vi "Read Set.vi"(8 "error in (no error)":errorcluster, 11 "VISA resource name":refnum<visa-resource-name>) -> (0 "error out":errorcluster, 1 "Set Current Level (A)":dbl format="%.2g", 2 "Set Voltage Level (V)":dbl format="%.2g", 3 "VISA resource name out":refnum<visa-resource-name>)   [LabVIEW 2017, in "ScientiFic DC Power Supply.lvlib"]
doc: "Returns the Set voltage level and Set current level for a desired channel."
uses:
  ScientiFic DC Power Supply.lvlib
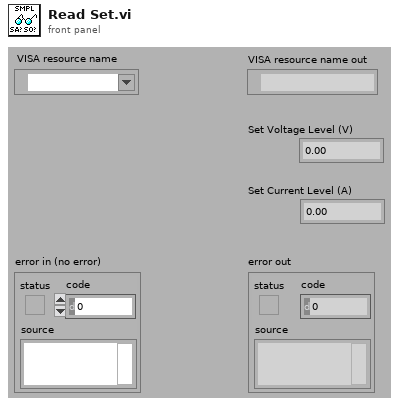
[diagram p1: front panel]
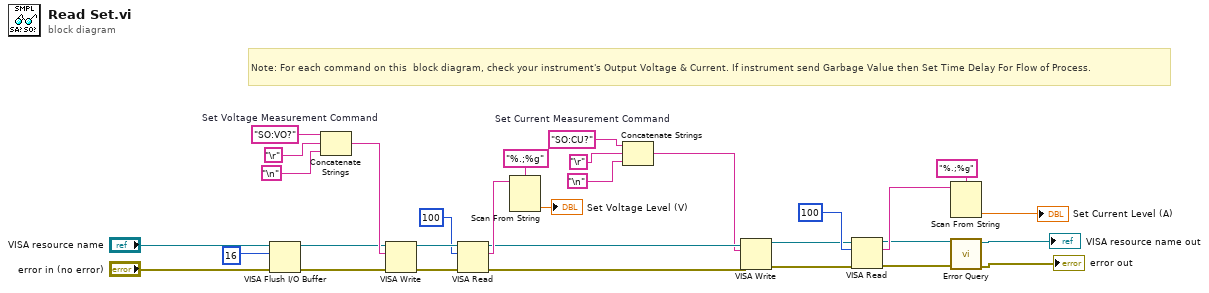
[diagram p0: block diagram]
diagram:
  w7 = "SO:CU?"  # Set Current Measurement Command
  w11 = "SO:VO?"  # Set Voltage Measurement Command
  # "Note: For each command on this  block diagram, check your instrument's Output Voltage & Current. If instrument send Garbage Value then Set Time Delay For Flow of Process."
  n1 = VISA Flush I/O Buffer(VISA resource name="VISA resource name", mask (16)=u16 16, error in (no error)="error in (no error)") -> (VISA resource name out=w4:refnum<visa-resource-name>, error out=w2:errorcluster)
  n2 = Concatenate Strings(w11, "\r", "\n") -> (w10:string)
  n3 = VISA Write(VISA resource name=w4, write buffer=w10, error in (no error)=w2) -> (VISA resource name out=w30:refnum<visa-resource-name>, error out=w31:errorcluster)  [unwired: 1 out]
  n4 = VISA Read(VISA resource name=w30, byte count=u32 100, error in (no error)=w31) -> (VISA resource name out=w14:refnum<visa-resource-name>, read buffer=w25:string, error out=w15:errorcluster)  [unwired: 1 out]
  n5 = Scan From String(format string="%.;%g", input string=w25) -> (output 1=→"Set Voltage Level (V)":dbl)  [unwired: 3 in, 3 out]
  n6 = Concatenate Strings(w7, "\r", "\n") -> (w6:string)
  n7 = VISA Write(VISA resource name=w14, write buffer=w6, error in (no error)=w15) -> (VISA resource name out=w20:refnum<visa-resource-name>, error out=w19:errorcluster)  [unwired: 1 out]
  n8 = VISA Read(VISA resource name=w20, byte count=u32 100, error in (no error)=w19) -> (VISA resource name out=w17:refnum<visa-resource-name>, read buffer=w22:string, error out=w16:errorcluster)  [unwired: 1 out]
  n9 = Scan From String(format string="%.;%g", input string=w22) -> (output 1=→"Set Current Level (A)":dbl)  [unwired: 3 in, 3 out]
  n10 = call "Error Query.vi"("error in (no error)"=w16, "VISA resource name"=w17) -> ("error out"=→"error out":errorcluster, "VISA resource name out"=→"VISA resource name out":refnum<visa-resource-name>)  [unwired: 8 in]
